vi "query pattern.vi"() -> ()   [LabVIEW 2025]
uses:
  <instrlib>/Chroma 19052/Chroma 19052.lvlib
panel:
  out "error out":errorcluster
  in  "error in (no error)":errorcluster
  out "VISA resource name out":refnum<visa-resource-name>
  in  "VISA resource name":refnum<visa-resource-name>
  out "Result":string
  in  "Step":u8=1 min=1 max=99 step=1
  # "query"
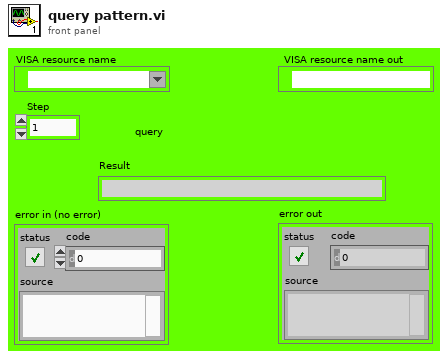
[diagram p1: front panel]
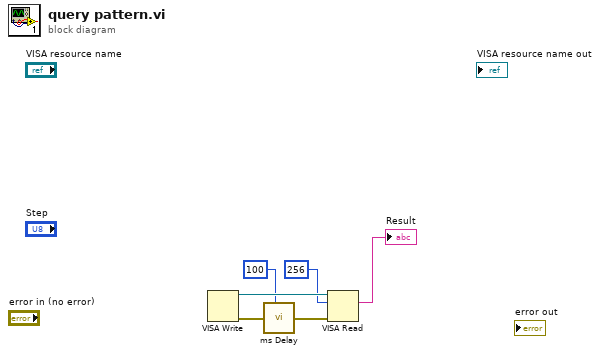
[diagram p0: block diagram]
diagram:
  n1 = VISA Write() -> (VISA resource name out=w6:refnum<visa-resource-name>, error out=w5:errorcluster)  [unwired: 3 in, 1 out]
  n2 = call <instrlib>:"ms Delay.vi"("miliseconds to wait"=u32 100 ("Time Delay ms"), "error in (no error)"=w5) -> ("error out"=w4:errorcluster)  [unwired: 6 in, 1 out]
  n3 = VISA Read(VISA resource name=w6, byte count=u32 256, error in (no error)=w4) -> (read buffer=→"Result":string)  [unwired: 3 out]
